vi "Complex Number to String (CSG).vi"(1 "use system decimal point (T)":bool=TRUE, 2 "precision (6)":i16, 3 "width (-)":i16, 4 "number":csg) -> (0 "Complex-format string":string)   [LabVIEW 2018, in "Numeric Data Type.lvclass"]
doc: "<b> </b> <b> </b>\n©2013, Q Software Innovations, LLC.\n\nWritten in National Instruments LabVIEW™ 2013.\n\nAuthored by Quentin Alldredge\nQ@qsoftwareinnovations.com\nwww.qsoftwareinnovations.com\n\nAll rights reserved."
uses:
  Numeric Data Type.lvclass
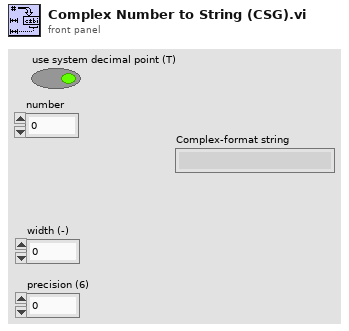
[diagram p1: front panel]
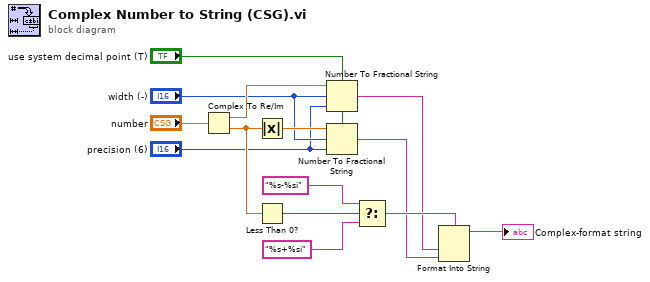
[diagram p0: block diagram]
diagram:
  n1 = Complex To Re/Im(x + iy="number") -> (x=w13:sgl, y=w12:sgl)
  n2 = Absolute Value(x=w12) -> (abs(x)=w11:sgl)
  n3 = Less Than 0?(x=w12) -> (x < 0?=w10:bool)
  n4 = Number To Fractional String(use system decimal point (T)="use system decimal point (T)", number=w13, width (-)="width (-)", precision (6)="precision (6)") -> (F-format string=w5:string)
  n5 = Number To Fractional String(use system decimal point (T)="use system decimal point (T)", number=w11, width (-)="width (-)", precision (6)="precision (6)") -> (F-format string=w4:string)
  n6 = Select(t="%s-%si", s=w10, f="%s+%si") -> (s? t:f=w6:string)
  n7 = Format Into String(format string=w6, w5, w4) -> (resulting string=→"Complex-format string":string)  [unwired: 2 in, 1 out]
